vi "Start Config.vi"(8 "error in":errorcluster, 11 "cPAS in":refnum<class "cPAS.lvclass">) -> (0 "error out":errorcluster, 3 "cPAS out":refnum<class "cPAS.lvclass">)   [LabVIEW 2015, in "cPAS.lvclass"]
doc: "Perform configuration of cells and data classes as well as switching and anything else that might not fit into the other config VIs. This VI can be used to set up a single cell with the default PAS Data Class, PAS Cell class, and a speaker switch setting of firing every 5 minutes for 1 second."
uses:
  cPAS.lvclass
  Devices/TE Cooler/TE Cooler.lvclass
  Reusable/Session APIs/File Access/Config Data/Config Data.lvclass
  Reusable/Session APIs/Serial/Serial Session.lvclass
  Reusable/Session APIs/File Access/Config Data/Config Session.ctl
  Reusable/Session Log/System Log.lvclass
  Reusable/Session APIs/File Access/Config Data/Config Data.lvclass/Config Data.ctl
  cPAS.lvclass/cPAS.ctl
  Reusable/Session Log/System Log.lvclass/System Log.ctl
  Reusable/Session APIs/Text Communication/Text Device Session.lvclass/Text Device Session.ctl
  Devices/Configurable Device/Configurable Device.lvclass/Configurable Device.ctl
  Devices/TE Cooler/TE Cooler.lvclass/TE Cooler.ctl
  Reusable/Session Log/Accessors/Write Main Path.vi
  Reusable/Session APIs/Text Communication/Write hSysLog.vi
  Devices/Configurable Device/Write Handle.vi
  Devices/TE Cooler/Write hSession.vi
  Devices/TE Cooler/Write ID.vi
  Reusable/PAS/Main/Read Switch Ref.vi
  Reusable/Switch/Read maxElapsedTime.vi
  Reusable/Switch/Switch.lvclass
  <userlib>/_Session Fwk/Session - Root.lvclass
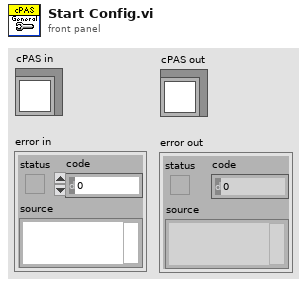
[diagram p1: front panel]
types:
  T1 = typedef "Config Data.lvclass/Config Session.ctl" = refnum<data-value>
  T2 = cluster{"Cell 1":sgl, "Cell 2":sgl, "Cell 3":sgl, "Cell 4":sgl, "Cell 5":sgl}
  T3 = cluster{"Cell 1":bool, "Cell 2":bool, "Cell 3":bool, "Cell 4":bool, "Cell 5":bool}
  T4 = typedef "Session - Root.lvclass/Session Handle.ctl" = refnum<data-value>
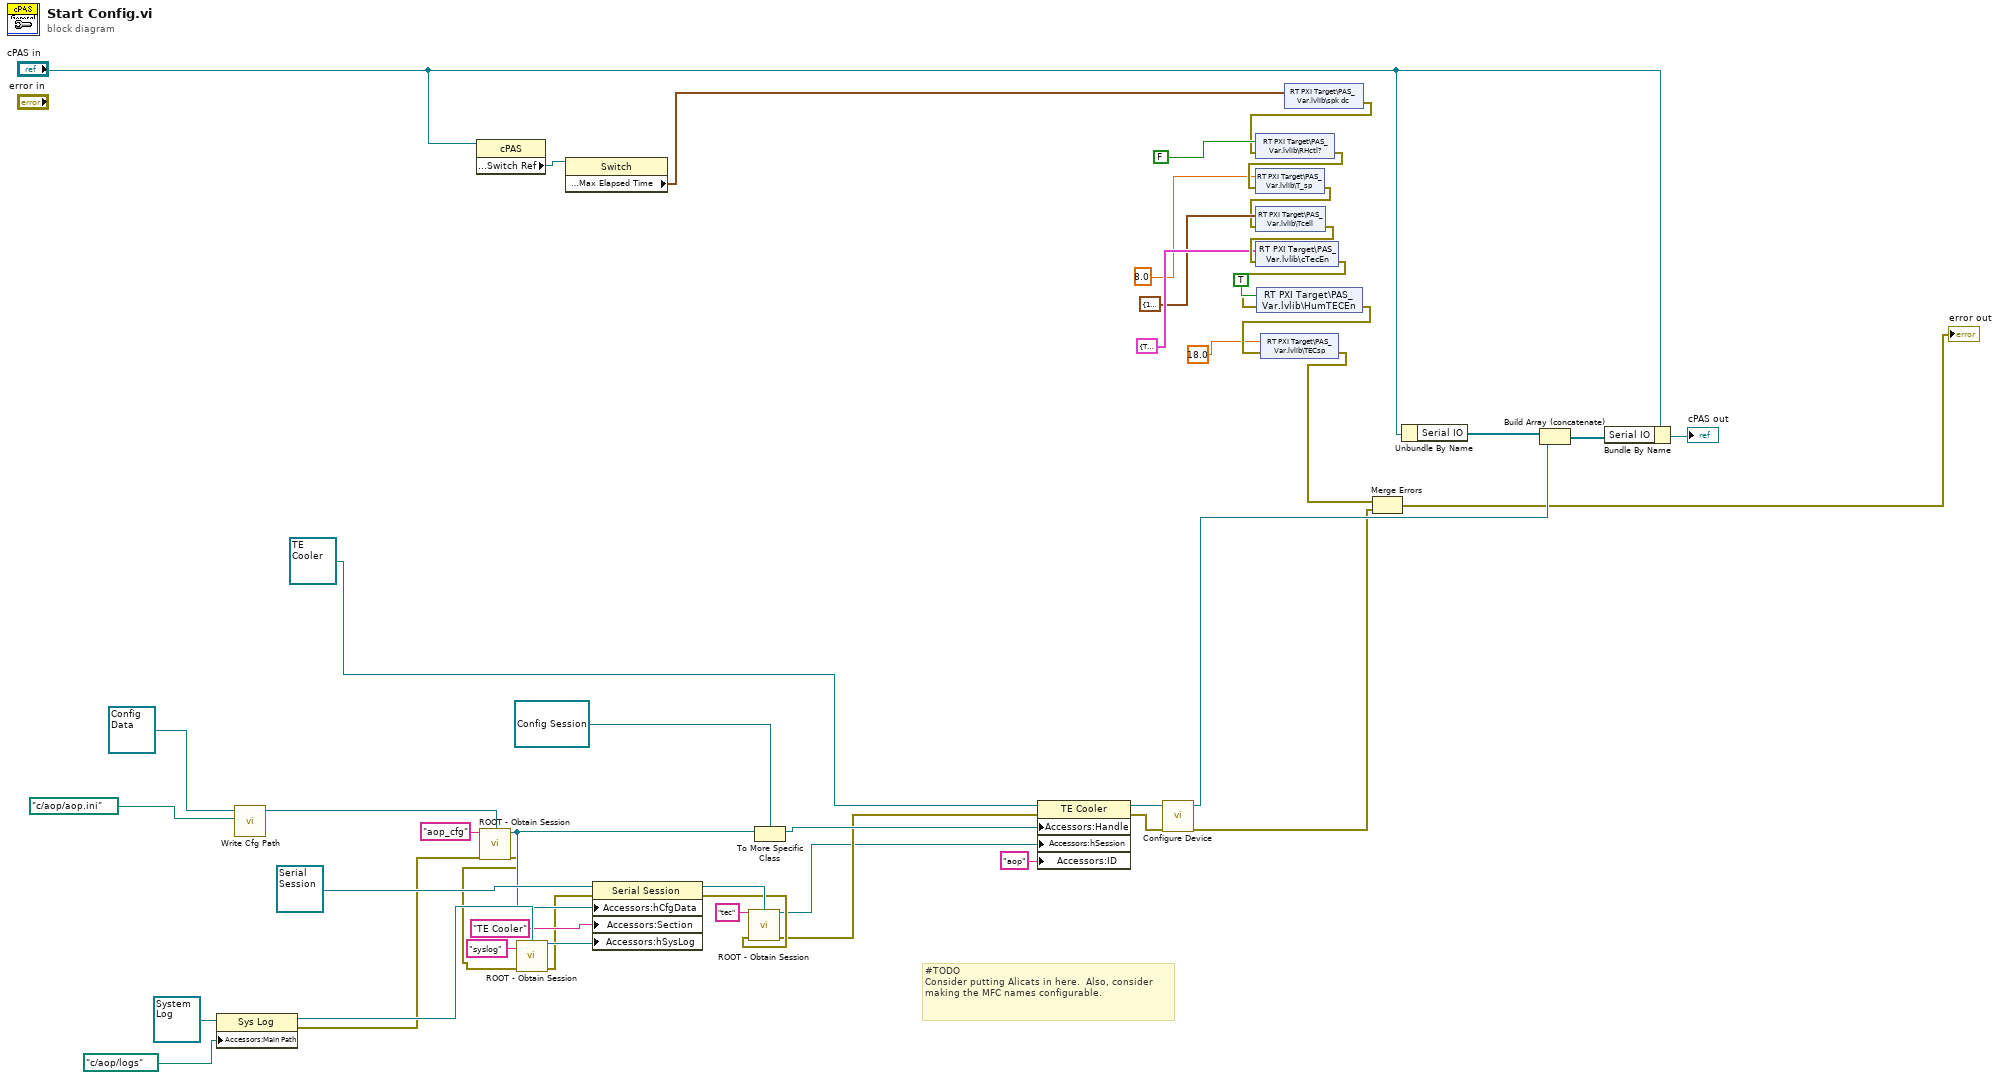
[diagram p0: block diagram]
diagram:
  # "#TODO\nConsider putting Alicats in here.  Also, consider making the MFC names configurable."
  n1 = property class="Sys Log"(reference=refnum<class "System Log.lvclass"> refnum ("Sys Log"), "Accessors:Main Path"=path "c:/aop/logs" ("Main Path")) -> (reference out=w26:refnum<class "System Log.lvclass">, error out=w25:errorcluster)  [unwired: 1 in]
  n2 = call "Write Cfg Path.vi"("Cfg Path"=path "c:/aop/aop.ini", "Config Data in"=refnum<class "Config Data.lvclass"> refnum ("Config Data")) -> ("Config Data out"=w32:refnum<class "Config Data.lvclass">)  [unwired: 8 in, 1 out]
  n3 = property class="cPAS"(reference="cPAS in") -> ("Data Access:Switch Ref"=w2:refnum<class "Switch.lvclass">)  [unwired: 1 in, 2 out]
  n4 = call <userlib>:"ROOT - Obtain Session.vi"("Session Name ()"="aop_cfg", "OBJ - Session"=w32, "error in (no error)"=w25) -> ("Session Handle"=w19:T4, "error out"=w13:errorcluster)  [unwired: 10 in, 1 out]
  n5 = call <userlib>:"ROOT - Obtain Session.vi"("Session Name ()"="syslog", "OBJ - Session"=w26, "error in (no error)"=w13) -> ("Session Handle"=w16:T4, "error out"=w12:errorcluster)  [unwired: 10 in, 1 out]
  n6 = property class="Switch"(reference=w2) -> ("Data Access:Max Elapsed Time"=w1:cluster{"true":sgl, "false":sgl})  [unwired: 1 in, 2 out]
  n7 = property class="Serial Session"(reference=refnum<class "Serial Session.lvclass"> refnum ("Serial Session"), error in=w12, "Accessors:hCfgData"=w19, "Accessors:Section"="TE Cooler" ("Section"), "Accessors:hSysLog"=w16) -> (reference out=w21:refnum<class "Serial Session.lvclass">, error out=w11:errorcluster)
  n8 = call <userlib>:"ROOT - Obtain Session.vi"("Session Name ()"="tec", "OBJ - Session"=w21, "error in (no error)"=w11) -> ("Session Handle"=w9:T4, "error out"=w10:errorcluster)  [unwired: 10 in, 1 out]
  n9 = To More Specific Class(target class=T1 refnum ("Handle"), reference=w19) -> (specific class reference=w18:T1)  [unwired: 1 in, 1 out]
  n10 = property class="TE Cooler"(reference=refnum<class "TE Cooler.lvclass"> refnum ("TE Cooler.lvlib:TE Cooler.lvclass"), error in=w10, "Accessors:Handle"=w18, "Accessors:hSession"=w9, "Accessors:ID"="aop" ("ID")) -> (reference out=w15:refnum<class "TE Cooler.lvclass">, error out=w14:errorcluster)
  n11 = call-dynamic "Configure Device.vi"("error in"=w14, "TE Cooler in"=w15) -> ("error out"=w5:errorcluster, "TE Cooler out"=w7:refnum<class "TE Cooler.lvclass">)  [unwired: 8 in]
  n12 = shared-variable "RT PXI Target\\PAS_Var.lvlib\\spk dc"(w1) -> (error out=w34:errorcluster)  [unwired: 1 in]
  n13 = shared-variable "RT PXI Target\\PAS_Var.lvlib\\RHctl?"(FALSE ("RH ctl"), error in=w34) -> (error out=w48:errorcluster)
  n14 = shared-variable "RT PXI Target\\PAS_Var.lvlib\\T_sp"(sgl 8.0 ("T"), error in=w48) -> (error out=w41:errorcluster)
  n15 = shared-variable "RT PXI Target\\PAS_Var.lvlib\\Tcell"(T2 {"Cell 1"=10.0, "Cell 2"=10.0, "Cell 3"=10.0, "Cell 4"=10.0, "Cell 5"=10.0} ("Tcell"), error in=w41) -> (error out=w47:errorcluster)
  n16 = shared-variable "RT PXI Target\\PAS_Var.lvlib\\cTecEn"(T3 {"Cell 1"=TRUE, "Cell 2"=TRUE, "Cell 3"=TRUE, "Cell 4"=TRUE, "Cell 5"=TRUE} ("cTecEn"), error in=w47) -> (error out=w40:errorcluster)
  n17 = shared-variable "RT PXI Target\\PAS_Var.lvlib\\HumTECEn"(TRUE ("HumTECEn"), error in=w40) -> (error out=w39:errorcluster)
  n18 = shared-variable "RT PXI Target\\PAS_Var.lvlib\\TECsp"(sgl 18.0 ("Data Access:TSP"), error in=w39) -> (error out=w6:errorcluster)
  n19 = Merge Errors(w6, w5) -> (→"error out":errorcluster)
  n20 = Unbundle By Name("cPAS in") -> ("Serial IO"=w38:refnum<class "Configurable Device.lvclass">[])
  n21 = Build Array (concatenate)(w38, w7) -> (w37:refnum<class "Configurable Device.lvclass">[])
  n22 = Bundle By Name(cluster="cPAS in", "Serial IO"=w37) -> (→"cPAS out":refnum<class "cPAS.lvclass">)
